vi "Attempt Connection.vi"(8 "error in (no error)":errorcluster, 11 "Connection Info":T1) -> (0 "error out":errorcluster, 3 "Connection Info (duplicate)":T1)   [LabVIEW 2020, in "plugin_flodx_ph_probe.lvlib" / "plugin.lvlib" / "Instrument Manager.lvlib"]
doc: "Attempt to connect to the hardware based on the connection info provided. The relevant error will be returned if the connection fails."
uses:
  Instrument Manager.lvlib
  connection_info/Connection Info.ctl
  mock_driver/mock_driver.lvlib
  <instrlib>/RxnRover/FloDx Ph Probe Driver/driver_flodx_ph_probe.lvlib
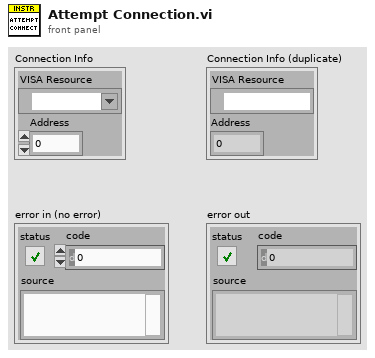
[diagram p1: front panel]
types:
  T1 = typedef "plugin_flodx_ph_probe.lvlib/plugin.lvlib/Instrument Manager.lvlib/Connection Info.ctl" = cluster{"VISA Resource":refnum<visa-resource-name>, "Address":u8}
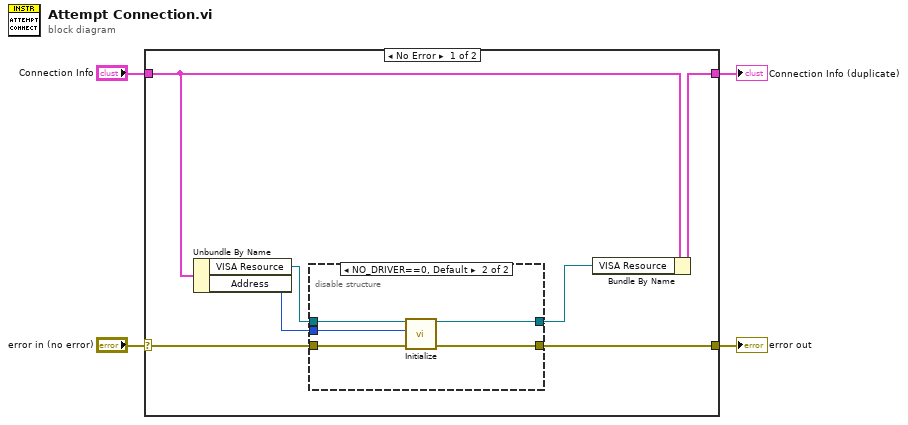
[diagram p0: block diagram]
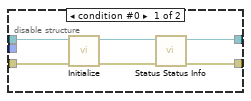
[diagram p2: hidden frame]
diagram:
  n1 = case shown="No Error" "error in (no error)" {
    selector: "error in (no error)" -> [w9 w23]
    tunnel: [w11 w23] -> w4
    tunnel: "Connection Info" -> [w8 w24]
    tunnel: [w7 w24] -> w1
    frame No Error {
      n2 = Unbundle By Name(w8) -> ("VISA Resource"=w10:refnum<visa-resource-name>, "Address"=w5:u8)
      n3 = disable-structure shown="NO_DRIVER==0, Default" {
        disable-tunnel: w9 -> [w17 w19]
        disable-tunnel: w10 -> [w15 w20]
        disable-tunnel: [w14 w22] -> w11
        disable-tunnel: [w12 w21] -> w6
        disable-tunnel: w5 -> [_ w18]
        frame condition #0 {
          n4 = call <instrlib>:"Initialize.vi"("Error in"=w17, "VISA resource name"=w15) -> ("Error out"=w16:errorcluster, "VISA resource name out"=w13:refnum<visa-resource-name>)  [unwired: 8 in]
          n5 = call "Status Status Info.vi"("error in (no error)"=w16, "VISA Resource in"=w13) -> ("error out"=w14:errorcluster, "VISA Resource out"=w12:refnum<visa-resource-name>)  [unwired: 6 in, 2 out]
        }
        frame condition #1 (active) {
          n6 = call <instrlib>:"Initialize.vi"("error in (no error)"=w19, "Address"=w18, "VISA resource name"=w20) -> ("error out"=w22:errorcluster, "VISA resource name out"=w21:refnum<visa-resource-name>)  [unwired: 6 in, 1 out]
        }
      }
      n7 = Bundle By Name(cluster=w8, "VISA Resource"=w6) -> (w7:T1)
    }
    frame Error {
    }
  }
  "error out" <- w4
  "Connection Info (duplicate)" <- w1
